vi "Vision Research Phantom Series PhFile PhGetCineImage.vi"(0 "hC [in]":u32=1, 1 "pRng [in]":T2, 2 "bufferByteSize [in]":u32, 3 "pPixelBuffer [in]":u16[](array[numeric]), 5 "Error In (no error)":errorcluster) -> (14 "hC [out]":u32, 15 "pPixelBuffer [out]":u16[](array[numeric]), 16 "IH [out]":T1, 19 "Error Out":errorcluster)   [LabVIEW 2013, in "VRI.lvlib"]
doc: "PhGetCineImage\nHRESULT PhGetCineImage(CINEHANDLE hC, PIMRANGE pRng, PBYTE pPixelBuffer,\n UINT bufferByteSize, PIH pIH)\n\nParameters\nhC [in]\n Cine to read images from.\npRng [in, optional]\n Requested image range.\n For live cines, this parameter is NULL.\npPixelBuffer [out]\n Buffer where to store requested image data.\nbufferByteSize [in]\n Buffer size in bytes.\npIH [out]\n Image header describing buffer image data.\n\nReturn Value\nThe function returns ERR_Ok in case of success or an error code, otherwise. To get extended error information call PhGetErrorMessage.\n\nRemarks\nReads and processes images from the input cine and stores them in pPixelBuffer buffer. The function can be used for any type of cine: live cine, camera cine or file cine. \nRequested images are read from the source cine and then processed according to current use case and corresponding parameters. See PhSetUseCase, PhGetUseCase for more details.\nThe image header, pIH, fully describes the final image format.\nUse pRng to specify what images you are interested in. For live cines, this parameter can be NULL, in which case the function will return one live image.\nThe pixel buffer, pPixelBuffer, is used for storing images all throughout the processing pipeline. For this reason, it must be large enough to accommodate all the images no matter the processing phase. To obtain the maximum memory size necessary for processing one image call PhSetCineInfo with the GCI_MAXIMGSIZE selector.\nNo more than one PhGetCineImage call per CINEHANDLE object must exist at any given time.\n\nRequired Header\nPhFile.h"
uses:
  VRI.lvlib
  _Type Defs/PHCon IMRANGE.ctl
  _Type Defs/PhInt IH.ctl
  _Type Defs/PhFile PhSetCineInfo.ctl
  Phantom DLLs/PhFile.Dll
panel:
  # "For instructions on the use of this VI, press Ctrl+H to display the help window and move the mouse over the icon, controls, and indicators"
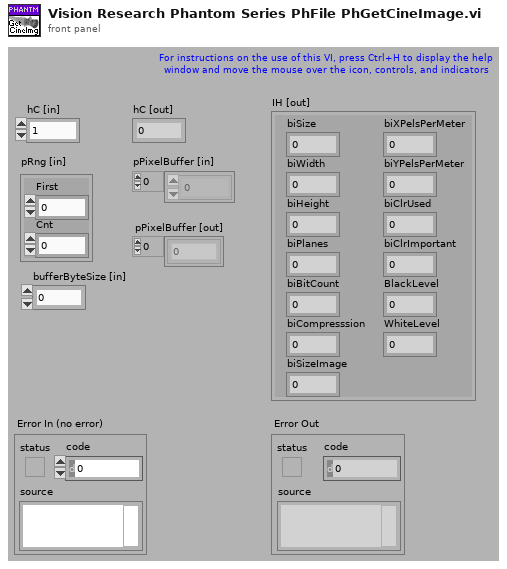
[diagram p1: front panel]
types:
  T1 = typedef "VRI.lvlib/PhInt IH.ctl" = cluster{"biSize":u32, "biWidth":i32, "biHeight":i32, "biPlanes":u16, "biBitCount":u16, "biCompresssion":u32, "biSizeImage":u32, "biXPelsPerMeter":i32, "biYPelsPerMeter":i32, "biClrUsed":u32, "biClrImportant":u32, "BlackLevel":i32, "WhiteLevel":i32}
  T2 = typedef "VRI.lvlib/PHCon IMRANGE.ctl" = cluster{"First":i32, "Cnt":u32}
  T3 = typedef "VRI.lvlib/PhFile PhSetCineInfo.ctl" = u32
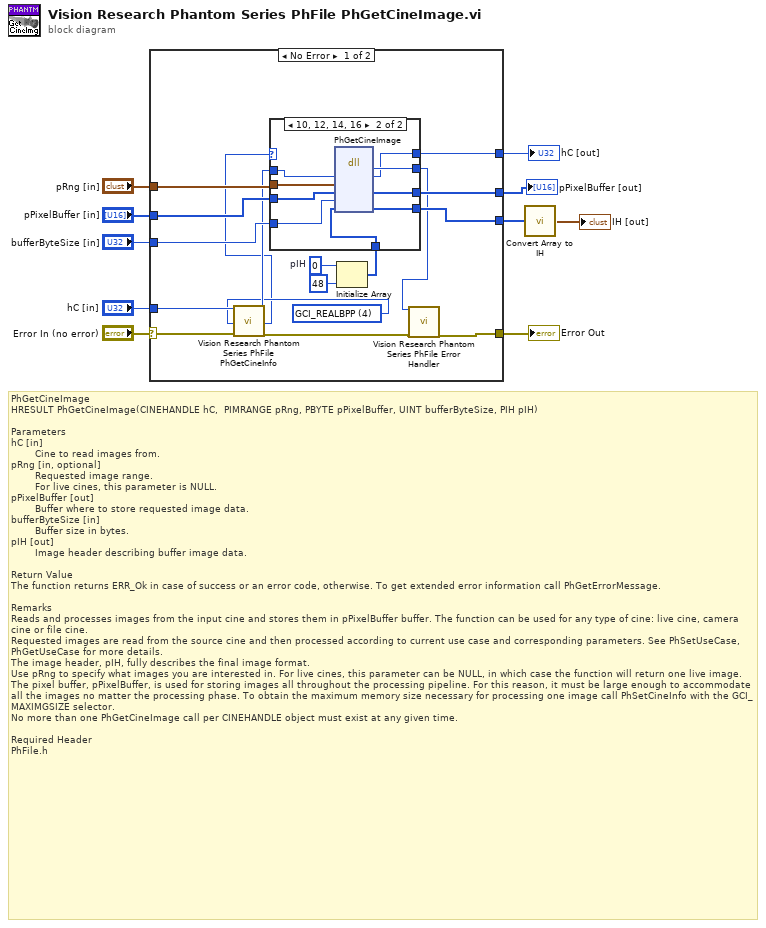
[diagram p0: block diagram]
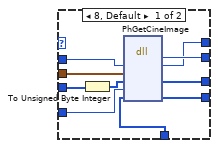
[diagram p2: hidden frame]
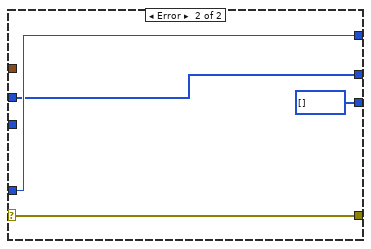
[diagram p3: hidden frame]
diagram:
  # "PhGetCineImage\nHRESULT PhGetCineImage(CINEHANDLE hC,  PIMRANGE pRng, PBYTE pPixelBuffer, UINT bufferByteSize, PIH pIH)\n\nParameters\nhC [in]\n        Cine to read images from.\npRng [in, optional]\n        Requested image range.\n        For live cines, this parameter is NULL.\npPixelBuffer [out]\n        Buffer where to store requested image data.\nbufferByteSize [in]\n        Buffer size in bytes.\npIH [out]\n        Image header describing buffer image data.\n\nReturn Value\nThe function returns ERR_Ok in case of success or an error code, otherwise. To get extended error information call PhGetErrorMessage.\n\nRemarks\nReads and processes images from the input cine and stores them in pPixelBuffer buffer. The function can be used for any type of cine: live cine, camera cine or file cine. \nRequested images are read from the source cine and then processed according to current use case and corresponding parameters. See PhSetUseCase, PhGetUseCase for more details.\nThe image header, pIH, fully describes the final image format.\nUse pRng to specify what images you are interested in. For live cines, this parameter can be NULL, in which case the function will return one live image.\nThe pixel buffer, pPixelBuffer, is used for storing images all throughout the processing pipeline. For this reason, it must be large enough to accommodate all the images no matter the processing phase. To obtain the maximum memory size necessary for processing one image call PhSetCineInfo with the GCI_MAXIMGSIZE selector.\nNo more than one PhGetCineImage call per CINEHANDLE object must exist at any given time.\n\nRequired Header\nPhFile.h"
  n1 = case shown="No Error" "Error In (no error)" {
    selector: "Error In (no error)" -> [w27 w50]
    tunnel: [w26 w50] -> w9
    tunnel: "hC [in]" -> [w25 w49]
    tunnel: "pRng [in]" -> [w24 _]
    tunnel: "bufferByteSize [in]" -> [w23 _]
    tunnel: [w22 u8[] [] ("pIH")] -> w2
    tunnel: "pPixelBuffer [in]" -> [w21 w48]
    tunnel: [w20 w48] -> w4
    tunnel: [w19 w49] -> w3
    frame No Error {
      w13 = u32 0  # pIH
      w17 = T3 4 items=["GCI_CFA"=0, "GCI_FRAMERATE"=1, "GCI_EXPOSURE"=2, "GCI_AUTOEXPOSURE"=3, "GCI_REALBPP"=4, "GCI_CAMERASERIAL"=5, "GCI_HEADSERIAL0"=6, "GCI_HEADSERIAL1"=7, "GCI_HEADSERIAL2"=8, "GCI_HEADSERIAL3"=9, "GCI_TRIGTIMESEC"=10, "GCI_TRIGTIMEFR"=11, "GCI_ISFILECINE"=12, "GCI_IS16BPPCINE"=13, "GCI_ISCOLORCINE"=14, "GCI_ISMULTIHEADCINE"=15, "GCI_EXPOSURENS"=16, "GCI_EDREXPOSURENS"=17, "GCI_FRAMEDELAYNS"=19, "GCI_FROMFILETYPE"=20, "GCI_COMPRESSION"=21, "GCI_CAMERAVERSION"=22, "GCI_ROTATE"=23, "GCI_IMWIDTH"=24, "GCI_IMHEIGHT"=25, "GCI_IMWIDTHACQ"=26, "GCI_IMHEIGHTACQ"=27, "GCI_POSTTRIGGER"=28, "GCI_IMAGECOUNT"=29, "GCI_TOTALIMAGECOUNT"=30, "GCI_TRIGFRAME"=31, "GCI_AUTOEXPLEVEL"=32, "GCI_AUTOEXPTOP"=33, "GCI_AUTOEXPLEFT"=34, "GCI_AUTOEXPBOTTOM"=35, "GCI_AUTOEXPRIGHT"=36, "GCI_RECORDINGTIMEZONE"=37, "GCI_FIRSTIMAGENO"=38, "GCI_FIRSTMOVIEIMAGE"=39, "GCI_CINENAME"=40, "GCI_FRPSTEPS"=100, "GCI_FRP1X"=101, "GCI_FRP1Y"=102, "GCI_FRP2X"=103, "GCI_FRP2Y"=104, "GCI_FRP3X"=105, "GCI_FRP3Y"=106, "GCI_FRP4X"=107, "GCI_FRP4Y"=108, "GCI_WRITEERR"=109, "GCI_LENSDESCRIPTION"=110, "GCI_LENSAPERATURE"=111, "GCI_LENSFOCALLENGTH"=112, "GCI_WB"=200, "GCI_WBVIEW"=201, "GCI_BRIGHT"=202, "GCI_CONTRAST"=203, "GCI_GAMMA"=204, "GCI_GAMMAR"=223, "GCI_GAMMAB"=224, "GCI_SATURATION"=205, "GCI_HUE"=206, "GCI_FLIPH"=207, "GCI_FLIPV"=208, "GCI_FILTERCODE"=209, "GCI_IMFILTER"=210, "GCI_INTALGO"=211, "GCI_PEDESTALR"=212, "GCI_PEDESTALG"=213, "GCI_PEDESTALB"=214, "GCI_FLARE"=225, "GCI_CHROMA"=226, "GCI_TONE"=227, "GCI_ENABLEMATRICES"=228, "GCI_USERMATRIX"=229, "GCI_RESAMPLEACTIVE"=215, "GCI_RESAMPLEWIDTH"=216, "GCI_RESAMPLEHEIGHT"=217, "GCI_CROPACTIVE"=218, "GCI_CROPRECTANGLE"=219, "GCI_OFFSET16_8"=220, "GCI_GAIN16_8"=221, "GCI_DEMOSAICINGFUNCPTR"=222, "GCI_VFLIPVIEWACTIVE"=300, "GCI_MAXIMGSIZE"=400, "GCI_FRPIMGNOARRAY"=450, "GCI_FRPRATEARRAY"=451, "GCI_FRPSHAPEARRAY"=452, "GCI_TRIGTC"=470, "GCI_TRIGTCU"=471, "GCI_PBRATE"=472, "GCI_TCRATE"=473, "GCI_SAVERANGE"=500, "GCI_SAVEFILENAME"=501, "GCI_SAVEFILETYPE"=502, "GCI_SAVE16BIT"=503, "GCI_SAVEPACKED"=504, "GCI_SAVEXML"=505, "GCI_SAVESTAMPTIME"=506, "GCI_SAVEAVIFRAMERATE"=520, "GCI_SAVEAVICOMPRESSORLIST"=521, "GCI_SAVEAVICOMPRESSORINDEX"=522, "GCI_SAVEDPXLSB"=530, "GCI_SAVEDPXTO10BPS"=531, "GCI_SAVEDPXDATAPACKING"=532, "GCI_SAVEDPX10BITLOG"=533, "GCI_SAVEDPXEXPORTLOGLUT"=534, "GCI_SAVEDPX10BITLOGREFWHITE"=535, "GCI_SAVEDPX10BITLOGREFBLACK"=536, "GCI_SAVEDPX10BITLOGGAMMA"=537, "GCI_SAVEDPX10BITLOGFILMGAMMA"=538, "GCI_SAVEQTPLAYBACKRATE"=550, "GCI_SAVECCIQUALITY"=560, "GCI_UNCALIBRATEDIMAGE"=600, "GCI_NOPROCESSING"=601, "GCI_BADPIXELREPAIR"=602]
      n2 = call "Vision Research Phantom Series PhFile PhGetCineInfo.vi"("CH in"=w25, "InfName"=w17, "Error In (no error)"=w27) -> ("CH out"=w18:u32, "pInfVal out"=w11:i32, "Error Out"=w16:errorcluster)  [unwired: 14 out]
      n3 = Initialize Array(w13, 48 ("dimension size")) -> (w12:u32[])
      n4 = case shown="10, 12, 14, 16" w11 {
        tunnel: w23 -> [w37 w42]
        tunnel: w21 -> [w31 w43]
        tunnel: w24 -> [w36 w45]
        tunnel: w18 -> [w35 w44]
        tunnel: [w34 w46] -> w15
        tunnel: [w33 w41] -> w22
        tunnel: [w29 w40] -> w20
        tunnel: [w32 w39] -> w19
        tunnel: w12 -> [w28 w38]
        frame 8, Default {
          n5 = To Unsigned Byte Integer(number=w31) -> (unsigned 8bit integer=w30:u8[])
          n6 = dll-call lib="C:/Projects/SDK/64-bit/Vision Research Phantom Series Labview Driver/Phantom DLLs/PhFile.dll" fn="PhGetCineImage"("hC"=w35, "pRng"=w36, "pPixelBuffer"=w30, "bufferByteSize"=w37, "pIH"=w28) -> ("HRESULT"=w34:i32, "hC"=w32:u32, "pPixelBuffer"=w29:u8[], "pIH"=w33:u8[])  [unwired: 5 in, 2 out]
        }
        frame 10, 12, 14, 16 {
          n7 = dll-call lib="C:/Projects/SDK/64-bit/Vision Research Phantom Series Labview Driver/Phantom DLLs/PhFile.dll" fn="PhGetCineImage"("hC"=w44, "pRng"=w45, "pPixelBuffer"=w43, "bufferByteSize"=w42, "pIH"=w38) -> ("HRESULT"=w46:i32, "hC"=w39:u32, "pPixelBuffer"=w40:u16[], "pIH"=w41:u8[])  [unwired: 5 in, 2 out]
        }
      }
      n8 = call "Vision Research Phantom Series PhFile Error Handler.vi"("Error Code (0)"=w15, "Error In (no error)"=w16) -> ("Error Out"=w26:errorcluster)  [unwired: 17 out]
    }
    frame Error {
    }
  }
  "Error Out" <- w9
  "pPixelBuffer [out]" <- w4
  "hC [out]" <- w3
  n9 = call "Convert Array to IH.vi"("Array"=w2) -> ("IH"=→"IH [out]":T1)
